vi "Phase Calculator v3.vi"(7 "error in (no error)":errorcluster, 8 "Feedback In":T1, 10 "Sensors":T2, 11 "Heel Strike?":bool) -> (0 "Feedkback Out":T1, 3 "Phase Angle (Phi)":dbl, 4 "error out":errorcluster)   [LabVIEW 2018]
uses:
  Sensor Data.ctl
  Phase Calculator Feedback Cluster.ctl
panel:
  out "Phase":dbl(graph)=-0.25043231955347145
  in  "Cluster":T1
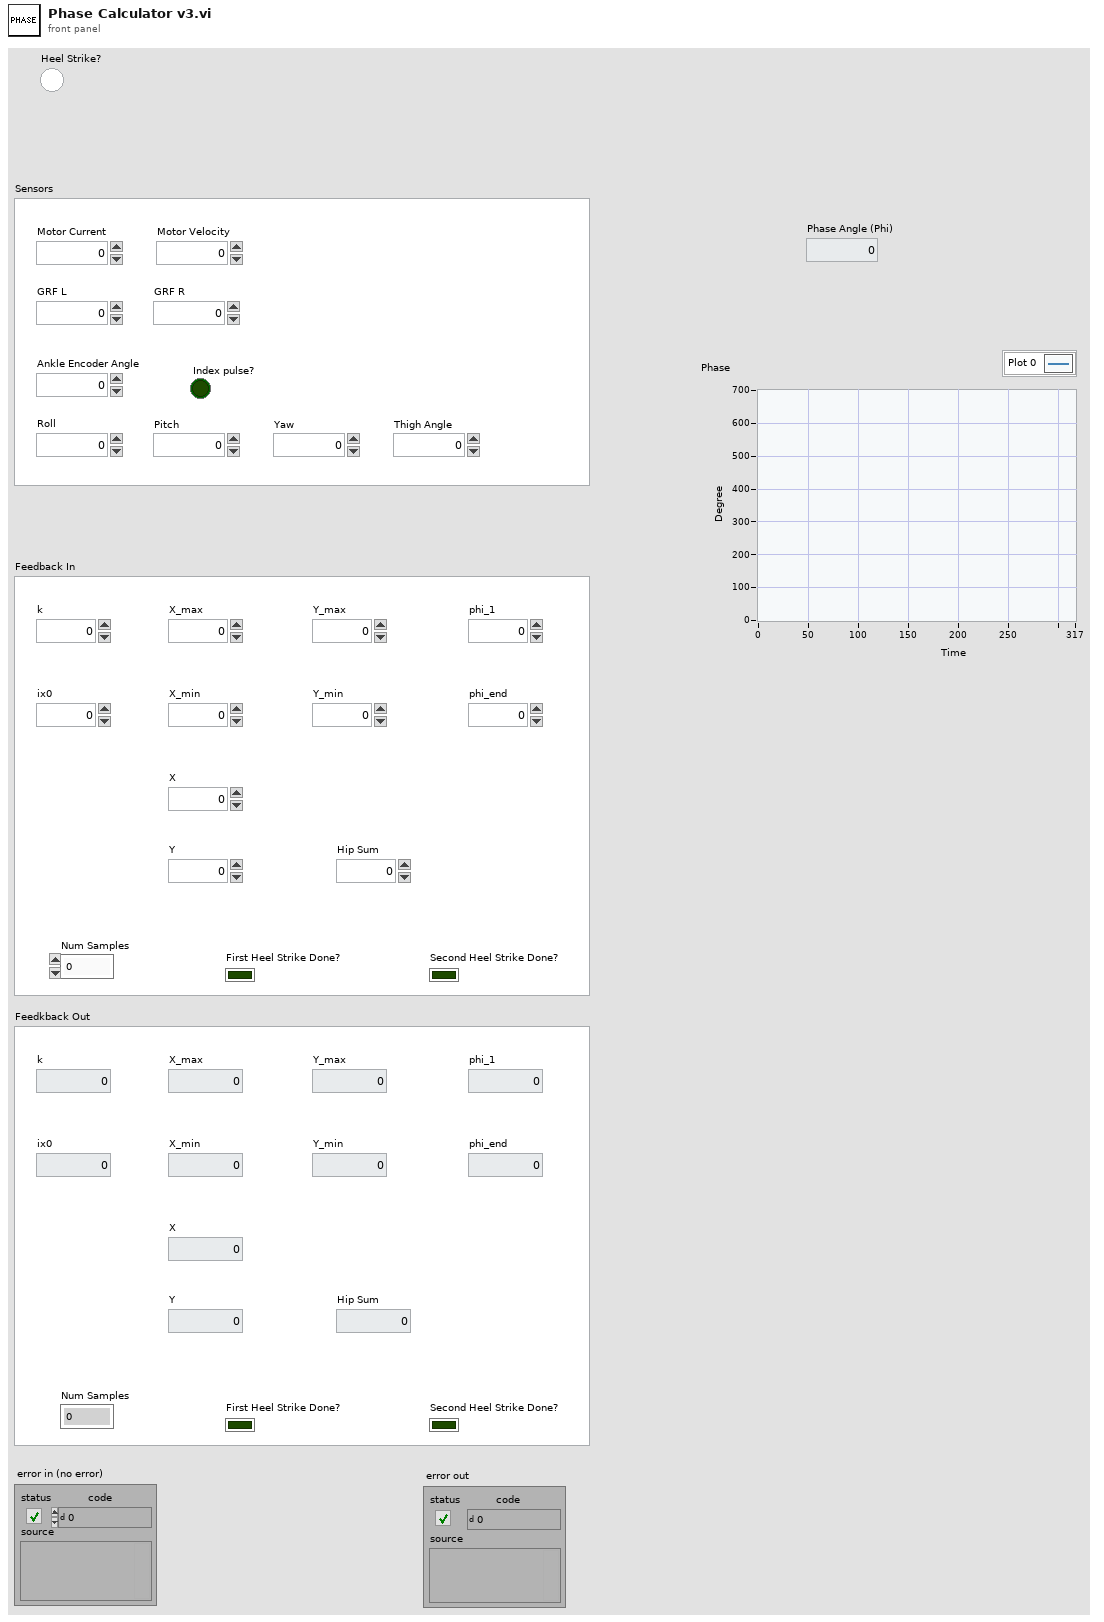
[diagram p1: front panel]
types:
  T1 = typedef "Phase Calculator Feedback Cluster.ctl" = cluster{"k":dbl, "ix0":dbl, "X_max":dbl, "X_min":dbl, "Y_max":dbl, "Y_min":dbl, "Y":dbl, "Hip Sum":dbl, "Num Samples":dbl, "First Heel Strike Done?":bool, "Second Heel Strike Done?":bool, "phi_1":dbl, "phi_end":dbl, "X":dbl}
  T2 = typedef "Sensor Data.ctl" = cluster{"Motor Current":dbl, "Motor Velocity":dbl, "Ankle Encoder Angle":dbl, "GRF L":dbl, "GRF R":dbl, "Index pulse?":bool, "Roll":dbl, "Pitch":dbl, "Yaw":dbl, "Thigh Angle":dbl}
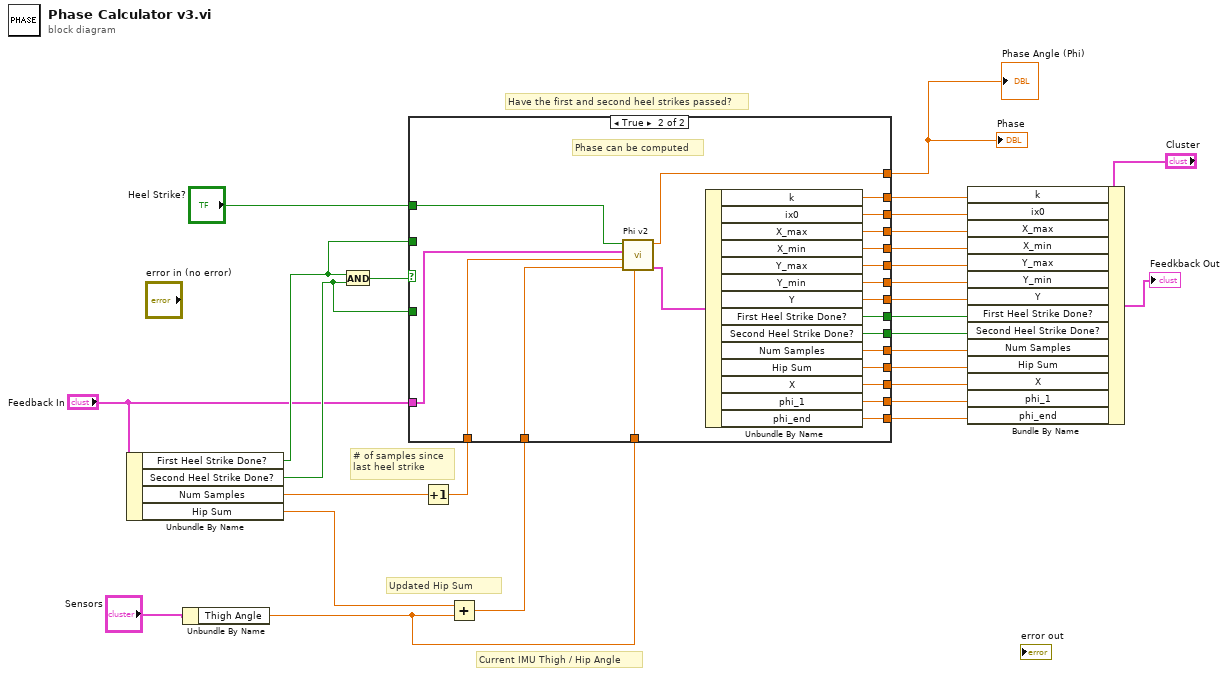
[diagram p0: block diagram]
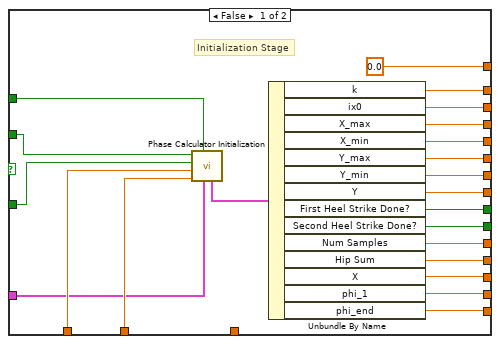
[diagram p2: hidden frame]
diagram:
  # "Current IMU Thigh / Hip Angle"
  # "Have the first and second heel strikes passed?"
  # "# of samples since \nlast heel strike"
  # "Updated Hip Sum"
  n1 = Unbundle By Name("Feedback In") -> ("First Heel Strike Done?"=w22:bool, "Second Heel Strike Done?"=w21:bool, "Num Samples"=w27:dbl, "Hip Sum"=w26:dbl)
  n2 = Unbundle By Name("Sensors") -> ("Thigh Angle"=w5:dbl)
  n3 = And(x=w22, y=w21) -> (x .and. y?=w23:bool)
  n4 = Increment(x=w27) -> (x+1=w18:dbl)
  n5 = Add(x=w26, y=w5) -> (x+y=w17:dbl)
  n6 = case shown="True" w23 {
    tunnel: w22 -> [w50 _]
    tunnel: w21 -> [w49 _]
    tunnel: "Heel Strike?" -> [w48 w71]
    tunnel: [0.0 w67] -> w4
    tunnel: "Feedback In" -> [w44 w70]
    tunnel: w18 -> [w46 w69]
    tunnel: w17 -> [w45 w68]
    tunnel: [w42 w65] -> w16
    tunnel: [w41 w64] -> w15
    tunnel: [w40 w63] -> w14
    tunnel: [w39 w62] -> w13
    tunnel: [w38 w61] -> w12
    tunnel: [w37 w60] -> w11
    tunnel: [w36 w59] -> w10
    tunnel: [w35 w58] -> w9
    tunnel: [w34 w57] -> w8
    tunnel: [w33 w56] -> w7
    tunnel: [w32 w55] -> w6
    tunnel: w5 -> [_ w54]
    tunnel: [w31 w53] -> w3
    tunnel: [w30 w52] -> w2
    tunnel: [w29 w51] -> w1
    frame False {
      # "Initialization Stage"
      n7 = call "Phase Calculator Initialization.vi"("Feedback In"=w44, "Heel Strike?"=w48, "Hip Sum"=w45, "Number of Samples"=w46, "HS2"=w49, "HS1"=w50) -> ("Feedback Out"=w43:T1)  [unwired: 5 in]
      n8 = Unbundle By Name(w43) -> ("k"=w42:dbl, "ix0"=w41:dbl, "X_max"=w40:dbl, "X_min"=w39:dbl, "Y_max"=w38:dbl, "Y_min"=w37:dbl, "Y"=w36:dbl, "First Heel Strike Done?"=w35:bool, "Second Heel Strike Done?"=w34:bool, "Num Samples"=w33:dbl, "Hip Sum"=w32:dbl, "X"=w31:dbl, "phi_1"=w30:dbl, "phi_end"=w29:dbl)
    }
    frame True {
      # "Phase can be computed"
      n9 = call "Phi v2.vi"("Current Hip Angle"=w54, "Hip  Sum"=w68, "Number of samples"=w69, "Feedback In"=w70, "Heel Strike?"=w71) -> ("Feedback Out"=w66:T1, "Phi"=w67:dbl)  [unwired: 5 in]
      n10 = Unbundle By Name(w66) -> ("k"=w65:dbl, "ix0"=w64:dbl, "X_max"=w63:dbl, "X_min"=w62:dbl, "Y_max"=w61:dbl, "Y_min"=w60:dbl, "Y"=w59:dbl, "First Heel Strike Done?"=w58:bool, "Second Heel Strike Done?"=w57:bool, "Num Samples"=w56:dbl, "Hip Sum"=w55:dbl, "X"=w53:dbl, "phi_1"=w52:dbl, "phi_end"=w51:dbl)
    }
  }
  "Phase Angle (Phi)" <- w4
  "Phase" <- w4
  n11 = Bundle By Name(cluster="Cluster", "k"=w16, "ix0"=w15, "X_max"=w14, "X_min"=w13, "Y_max"=w12, "Y_min"=w11, "Y"=w10, "First Heel Strike Done?"=w9, "Second Heel Strike Done?"=w8, "Num Samples"=w7, "Hip Sum"=w6, "X"=w3, "phi_1"=w2, "phi_end"=w1) -> (→"Feedkback Out":T1)
